vi "Read Measurement (Math).vi"(8 "error in (no error)":errorcluster, 9 "Timeout (10000 ms)":i32=10000, 11 "VISA resource name":refnum<visa-resource-name>) -> (0 "error out":errorcluster, 2 "Measurement":dbl, 3 "VISA resource name out":refnum<visa-resource-name>)   [LabVIEW 2019, in "Pendulum CNT90.lvlib"]
doc: "Reads data calculated in the post processing block. Use this VI to read the calculated or mathematics result."
uses:
  Pendulum CNT90.lvlib
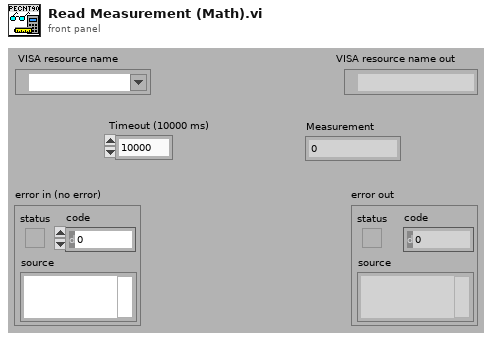
[diagram p1: front panel]
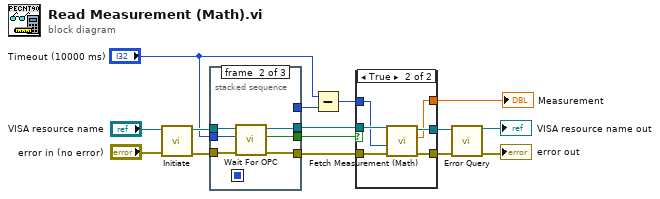
[diagram p0: block diagram]
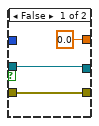
[diagram p2: hidden frame]
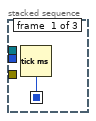
[diagram p3: hidden frame]
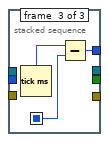
[diagram p4: hidden frame]
diagram:
  n1 = call "Initiate.vi"("error in (no error)"="error in (no error)", "VISA resource name"="VISA resource name") -> ("error out"=w7:errorcluster, "VISA resource name out"=w8:refnum<visa-resource-name>)  [unwired: 8 in]
  n2 = stacked-sequence {
    seq-local: [w16 _ _] -> [_ _ w24]
    tunnel: w8 -> [_ w19 _]
    tunnel: w7 -> [_ w20 _]
    tunnel: [_ w21 _] -> w5
    tunnel: [_ w22 _] -> w6
    tunnel: [_ _ w23] -> w3
    tunnel: [_ w18 _] -> w4
    tunnel: "Timeout (10000 ms)" -> [_ w17 _]
    frame #0 {
      n3 = Tick Count (ms)() -> (millisecond timer value=w16:u32)
    }
    frame #1 {
      n4 = call "Wait For OPC.vi"("error in (no error)"=w20, "Timeout (10000 ms)"=w17, "VISA resource name"=w19) -> ("error out"=w21:errorcluster, "Complete"=w18:bool, "VISA resource name out"=w22:refnum<visa-resource-name>)  [unwired: 6 in]
    }
    frame #2 {
      n5 = Tick Count (ms)() -> (millisecond timer value=w25:u32)
      n6 = Subtract(x=w25, y=w24) -> (x-y=w23:u32)
    }
  }
  n7 = Subtract(x="Timeout (10000 ms)", y=w3) -> (x-y=w1:u32)
  n8 = case shown="True" w4 {
    tunnel: [w28 w34] -> w11
    tunnel: [w27 w33] -> w10
    tunnel: [0.0 ("Data Result") w32] -> w9
    tunnel: w6 -> [w28 w31]
    tunnel: w5 -> [w27 w30]
    tunnel: w1 -> [_ w29]
    frame False {
    }
    frame True {
      n9 = call "Fetch Measurement (Math).vi"("error in (no error)"=w30, "Timeout (10000 ms)"=w29, "VISA resource name"=w31) -> ("error out"=w33:errorcluster, "Measurement"=w32:dbl, "VISA resource name out"=w34:refnum<visa-resource-name>)  [unwired: 6 in]
    }
  }
  "Measurement" <- w9
  n10 = call "Error Query.vi"("error in (no error)"=w10, "VISA resource name"=w11) -> ("error out"=→"error out":errorcluster, "VISA resource name out"=→"VISA resource name out":refnum<visa-resource-name>)  [unwired: 6 in, 2 out]
